vi "Acquisition trigger task-Create.vi"(8 "error in (no error)":errorcluster) -> (0 "error out":errorcluster, 3 "Acq. trigger task cluster":T1={"Encoder trigger AO task"="", "AO rate (Hz)"=1000000.0, "Encoder trigger pulse width (us)"=100.0})   [LabVIEW 2020]
uses:
  Typedefs/Trigger task cluster.ctl
  <vilib>/DAQmx/create/channels.llb/DAQmx Create Channel (CO-Pulse Generation-Time).vi
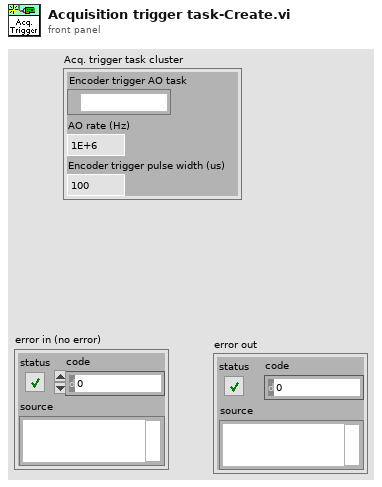
[diagram p1: front panel]
types:
  T1 = typedef "Trigger task cluster.ctl" = cluster{"Encoder trigger AO task":refnum<k21>, "AO rate (Hz)":dbl, "Encoder trigger pulse width (us)":dbl}
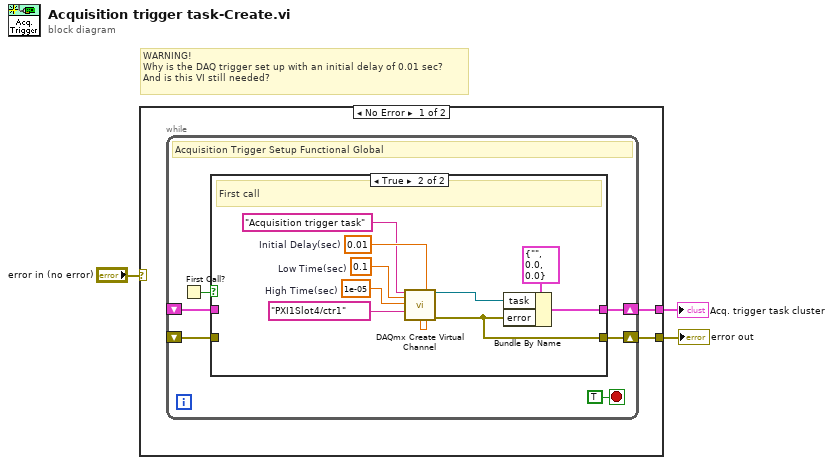
[diagram p0: block diagram]
diagram:
  # "WARNING!\nWhy is the DAQ trigger set up with an initial delay of 0.01 sec?\nAnd is this VI still needed?"
  n1 = case shown="No Error" "error in (no error)" {
    selector: "error in (no error)" -> [_ w23]
    tunnel: [w5 _] -> w3
    tunnel: [w4 w23] -> w2
    frame No Error {
      n2 = while {
        shift-right: [w11] -> w5
        shift-left: _ -> [w8]
        shift-right: [w7] -> w4
        shift-left: _ -> [w6]
        stop <- TRUE stop-if-true
        # "Acquisition Trigger Setup Functional Global"
        n3 = First Call?() -> (First Call?: T/F=w10:bool)
        n4 = case shown="True" w10 {
          tunnel: [w13 w22] -> w11
          tunnel: w8 -> [w13 _]
          tunnel: [w12 w15] -> w7
          tunnel: w6 -> [w12 _]
          frame False {
          }
          frame True {
            w18 = 0.01  # Initial Delay(sec)
            w20 = 0.1  # Low Time(sec)
            w19 = 1e-05  # High Time(sec)
            # "First call"
            n5 = call-poly <vilib>:"DAQmx Create Virtual Channel.vi"("task in"="Acquisition trigger task", "high time"=w19, "low time"=w20, "counter"=tag "PXI1Slot4/ctr1" ("DAQmx Digital Channel"), "initial delay"=w18) -> ("task out"=w16:refnum<k21>, "error out"=w15:errorcluster)  [unwired: 9 in]
            n6 = Bundle By Name(cluster=T1 {"Encoder trigger AO task"="", "AO rate (Hz)"=0.0, "Encoder trigger pulse width (us)"=0.0} ("Encoder trigger task cluster"), "task"=w16, "error"=w15) -> (w22:T1)
          }
        }
      }
    }
    frame Error {
    }
  }
  "Acq. trigger task cluster" <- w3
  "error out" <- w2
